vi "dfd_Match Remaining Zeros and Poles.vi"(10 "remaining poles":cdb[](array[numeric]), 11 "remaining zeros":cdb[](array[numeric])) -> (3 "matched zeros and poles":cluster{cdb[], cdb[]}[](array[cluster]))   [LabVIEW 2017, in "NI_DigFilterLicensed.lvlib"]
uses:
  <vilib>/addons/Digital Filter Design/NI_DigFilterLicensed.lvlib
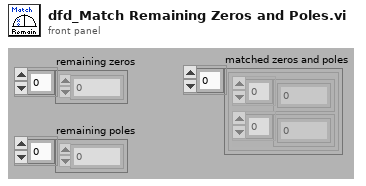
[diagram p1: front panel]
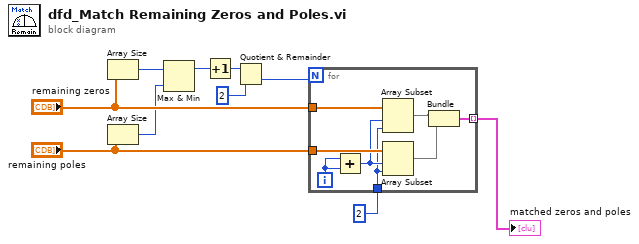
[diagram p0: block diagram]
diagram:
  n1 = Array Size(array="remaining zeros") -> (size(s)=w6:i32)
  n2 = Array Size(array="remaining poles") -> (size(s)=w1:i32)
  n3 = Max & Min(x=w6, y=w1) -> (max(x,y)=w2:i32)  [unwired: 1 out]
  n4 = Increment(x=w2) -> (x+1=w7:i32)
  n5 = Quotient & Remainder(x=w7, y=2) -> (floor(x/y)=w9:i32)  [unwired: 1 out]
  n6 = for {
    N: w9 -> [_]
    tunnel: "remaining zeros" -> [w18]
    tunnel: "remaining poles" -> [w17]
    tunnel: [w12] -> w10 mode=indexing
    tunnel: 2 ("y") -> [w11]
    i -> [w15]
    n7 = Add(x=w15, y=w15) -> (x+y=w16:i32)
    n8 = Array Subset(array=w18, index=w16, length=w11) -> (w14:cdb[])
    n9 = Array Subset(array=w17, index=w16, length=w11) -> (w13:cdb[])
    n10 = Bundle(w14, w13) -> (w12:cluster{cdb[], cdb[]})  [unwired: 1 out]
  }
  "matched zeros and poles" <- w10
